vi "Cond Init.vi"(8 "error in (no error)":errorcluster, 10 "Cond Attr in":T2, 11 "Cond in":T1) -> (0 "error out":errorcluster, 2 "Cond Attr out":T2, 3 "Cond out":T1)   [LabVIEW 2013, in "Linux RT IPC.lvlib" / "POSIX Threads.lvlib" / "Cond.lvclass"]
doc: "Calls pthread_cond_init() on the pthread cond object encapsulated by Cond.\n\nThis VI initializes the cond object and sets its attributes using the attributes contained in the Cond Attr object.\n\nRefer to online POSIX documentation for more information."
uses:
  Cond.lvclass
  Controls/reference.ctl
  Cond Attr/Controls/reference.ctl
  Cond Attr/Cond Attr.lvclass
  POSIX Thread Object/POSIX Thread Object.lvclass/POSIX Thread Object.ctl
  Cond.lvclass/Cond.ctl
  POSIX Thread Object/Private VIs/libpthread path.vi
  POSIX Thread Object/Private VIs/get pthread error.vi
  POSIX Thread Object/POSIX Thread Object.lvclass
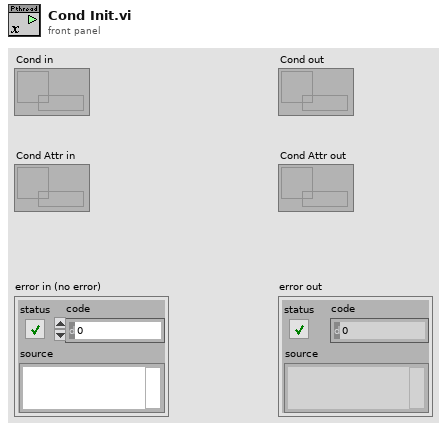
[diagram p1: front panel]
types:
  T1 = typedef "Linux RT IPC.lvlib/POSIX Threads.lvlib/Cond.lvclass/reference.ctl" = refnum<data-value>
  T2 = typedef "Linux RT IPC.lvlib/POSIX Threads.lvlib/Cond Attr.lvclass/reference.ctl" = refnum<data-value>
  T3 = typedef "Linux RT Utilities.lvlib/clockid_t.ctl" = enum16{"Realtime", "Monotonic"}
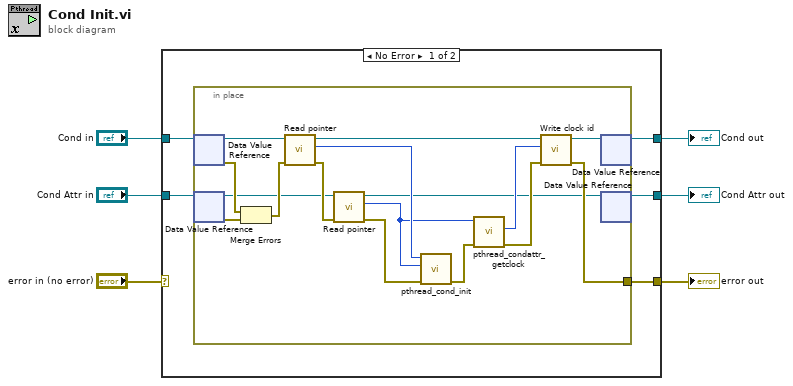
[diagram p0: block diagram]
diagram:
  n1 = case shown="No Error" "error in (no error)" {
    selector: "error in (no error)" -> [_ w30]
    tunnel: [w8 w30] -> w6
    tunnel: [w11 w28] -> w5
    tunnel: "Cond Attr in" -> [w10 w29]
    tunnel: [w9 w29] -> w3
    tunnel: "Cond in" -> [w7 w28]
    frame No Error {
      n2 = in-place {
        in-place-border: [w13] -> w8
        n3 = in-place-dvr #1(w7) -> (w27:refnum<class "Cond.lvclass">, w25:errorcluster)
        n4 = in-place-dvr #2(w10) -> (w22:refnum<class "Cond Attr.lvclass">, w26:errorcluster)
        n5 = Merge Errors(w25, w26) -> (w24:errorcluster)
        n6 = call "Read pointer.vi"("error in (no error)"=w24, "POSIX Thread Object in"=w27) -> ("error out"=w23:errorcluster, "pointer"=w18:u64, "POSIX Thread Object out"=w20:refnum<class "Cond.lvclass">)  [unwired: 7 in]
        n7 = call "Read pointer.vi"("error in (no error)"=w23, "POSIX Thread Object in"=w22) -> ("error out"=w21:errorcluster, "pointer"=w16:u64, "POSIX Thread Object out"=w12:refnum<class "Cond Attr.lvclass">)  [unwired: 7 in]
        n8 = call "pthread_cond_init.vi"("error in (no error)"=w21, "cond attr ptr in"=w16, "cond ptr in"=w18) -> ("error out"=w17:errorcluster)  [unwired: 6 in, 2 out]
        n9 = call "pthread_condattr_getclock.vi"("error in (no error)"=w17, "cond attr ptr in"=w16) -> ("error out"=w14:errorcluster, "clock id"=w15:T3)  [unwired: 7 in, 1 out]
        n10 = call "Write clock id.vi"("error in (no error)"=w14, "lv_clockid_t"=w15, "Cond in"=w20) -> ("error out"=w13:errorcluster, "Cond out"=w19:refnum<class "Cond.lvclass">)  [unwired: 7 in]
        n11 = in-place-dvr #1(w19) -> (w11:T1)  [unwired: 1 out]
        n12 = in-place-dvr #2(w12) -> (w9:T2)  [unwired: 1 out]
      }
    }
    frame Error {
    }
  }
  "Cond out" <- w5
  "error out" <- w6
  "Cond Attr out" <- w3
